vi "Speed graph cursor control.vi"(6 "Frame number":i32, 8 "error in (no error)":errorcluster, 9 "Initial frame":bool, 10 "Speed graph behaviour":T1, 11 "Speed graph ref":refnum<vi>) -> (0 "error out":errorcluster)   [LabVIEW 2013]
uses:
  Typedefs/Speed graph behaviour enum.ctl
  Globals/gl_Time series viewer globals.vi
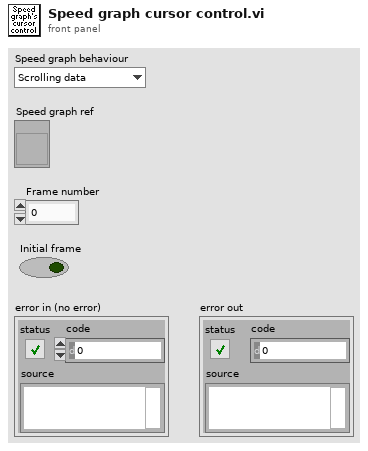
[diagram p1: front panel]
types:
  T1 = typedef "Speed graph behaviour enum.ctl" = enum16{"Scrolling data", "Scrolling cursor"}
  T2 = cluster{"Start Frame No":i32, "End Frame No":i32}
  T3 = typedef "Timelapse viewer refs.ctl" = cluster{"This VI":refnum<vi>, "AVI Mode ind":refnum<vi>, "Play":refnum<vi>, "Stop":refnum<vi>, "Back":refnum<vi>, "Scrollbar":refnum<vi>, "Video length info":refnum<vi>, "Expected speed values":refnum<vi>, "Intensity":refnum<vi>, "Path":refnum<vi>, "Selection sliders":refnum<vi>, "Speed Graph ref":refnum<vi>, "Frame rate set (fps)":refnum<vi>}
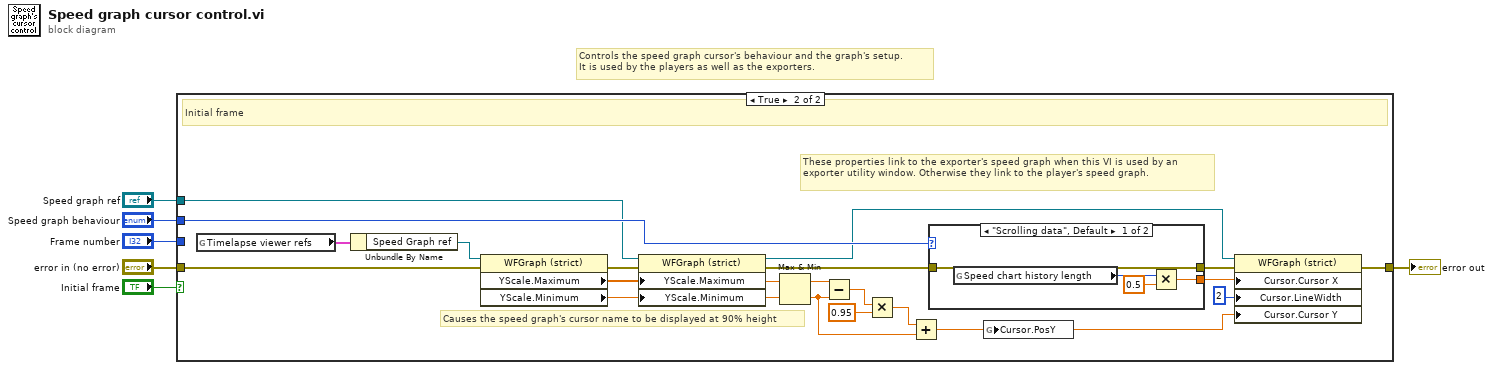
[diagram p0: block diagram]
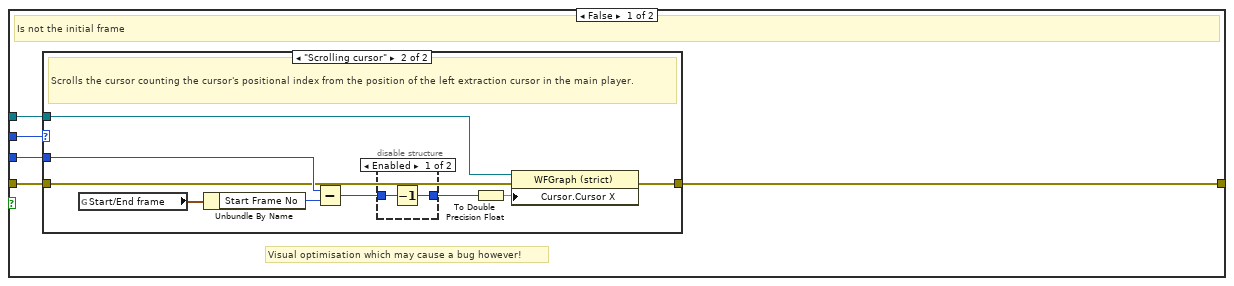
[diagram p2: hidden frame]
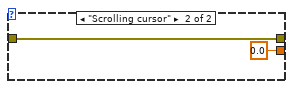
[diagram p5: hidden frame]
diagram:
  # "Controls the speed graph cursor's behaviour and the graph's setup.\nIt is used by the players as well as the exporters."
  n1 = case shown="True" "Initial frame" {
    tunnel: "Frame number" -> [w11 _]
    tunnel: "Speed graph behaviour" -> [w10 w44]
    tunnel: "Speed graph ref" -> [w9 w34]
    tunnel: [w8 w38] -> w4
    tunnel: "error in (no error)" -> [w7 w37]
    frame False {
      # "Visual optimisation which may cause a bug however!"
      # "Is not the initial frame"
      n2 = case shown="\"Scrolling cursor\"" w10 {
        tunnel: w11 -> [_ w19]
        tunnel: w9 -> [_ w17]
        tunnel: [w12 w16] -> w8
        tunnel: w7 -> [w12 w15]
        frame "Scrolling data", Default {
        }
        frame "Scrolling cursor" {
          # "Scrolls the cursor counting the cursor's positional index from the position of the left extraction cursor in the main player."
          n3 = global read "gl_Time series viewer globals.vi" "Start/End frame"() -> (w14:T2)
          n4 = Unbundle By Name(w14) -> ("Start Frame No"=w21:i32)
          n5 = Subtract(x=w19, y=w21) -> (x-y=w18:i32)
          n6 = disable-structure shown="Enabled" {
            disable-tunnel: w18 -> [w23 w24]
            disable-tunnel: [w22 w24] -> w13
            frame Enabled {
              n7 = Decrement(x=w23) -> (x-1=w22:i32)
            }
            frame Disabled {
            }
          }
          n8 = To Double Precision Float(number=w13) -> (double precision float=w20:dbl)
          n9 = property on="Property Node" class="WFGraph (strict)"(reference=w17, error in=w15, "Cursor.Cursor X"=w20) -> (error out=w16:errorcluster)  [unwired: 1 out]
        }
      }
    }
    frame True {
      # "Causes the speed graph's cursor name to be displayed at 90% height"
      # "These properties link to the exporter's speed graph when this VI is used by an exporter utility window. Otherwise they link to the player's speed graph."
      # "Initial frame"
      n10 = global read "gl_Time series viewer globals.vi" "Timelapse viewer refs"() -> (w42:T3)
      n11 = Unbundle By Name(w42) -> ("Speed Graph ref"=w43:refnum<vi>)
      n12 = property on="Property Node" class="WFGraph (strict)"(reference=w43, error in=w37) -> (error out=w36:errorcluster, "YScale.Maximum"=w32:dbl, "YScale.Minimum"=w31:dbl)  [unwired: 1 out]
      n13 = property on="Property Node" class="WFGraph (strict)"(reference=w34, error in=w36, "YScale.Maximum"=w32, "YScale.Minimum"=w31) -> (reference out=w33:refnum<vi>, error out=w35:errorcluster)
      n14 = Max & Min(x=w32, y=w31) -> (max(x,y)=w30:dbl, min(x,y)=w29:dbl)
      n15 = Subtract(x=w30, y=w29) -> (x-y=w28:dbl)
      n16 = Multiply(x=w28, y=0.95) -> (x*y=w27:dbl)
      n17 = Add(x=w27, y=w29) -> (x+y=w25:dbl)
      n18 = case shown="\"Scrolling data\", Default" w44 {
        tunnel: [w48 0.0] -> w41
        tunnel: w35 -> [w45 w49]
        tunnel: [w45 w49] -> w39
        frame "Scrolling data", Default {
          n19 = global read "gl_Time series viewer globals.vi" "Speed chart history length"() -> (w46:i32)
          n20 = Multiply(x=w46, y=0.5) -> (x*y=w48:dbl)
        }
        frame "Scrolling cursor" {
        }
      }
      n21 = global write "gl_Time series viewer globals.vi" "Cursor.PosY"(w25) -> ()
      n22 = property on="Property Node" class="WFGraph (strict)"(reference=w33, error in=w39, "Cursor.Cursor X"=w41, "Cursor.LineWidth"=u8 2 ("Cursor.Line Width"), "Cursor.Cursor Y"=w25) -> (error out=w38:errorcluster)  [unwired: 1 out]
    }
  }
  "error out" <- w4
